vi "Get VISA_Class.vi"(8 "error in":errorcluster, 9 "Sequence Context In":refnum<k7>, 10 "Config path":path=path "C:/GitHub/OOP_Submodule EOL/Config/INI Config.ini", 11 "Instrument":string="DMM") -> (0 "error out":errorcluster, 2 "Class":string, 3 "VISA Resource":string)   [LabVIEW 2021]
uses:
  Controls/Instrument.ctl
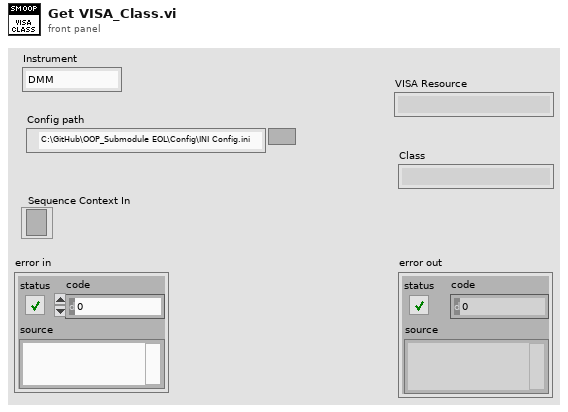
[diagram p1: front panel]
types:
  T1 = typedef "Instrument.ctl" = cluster{"Alias":string, "VISA Resource":string, "Class":string}
  T2 = typedef "MsgData.ctl" = cluster{"Message":string, "Data":variant}
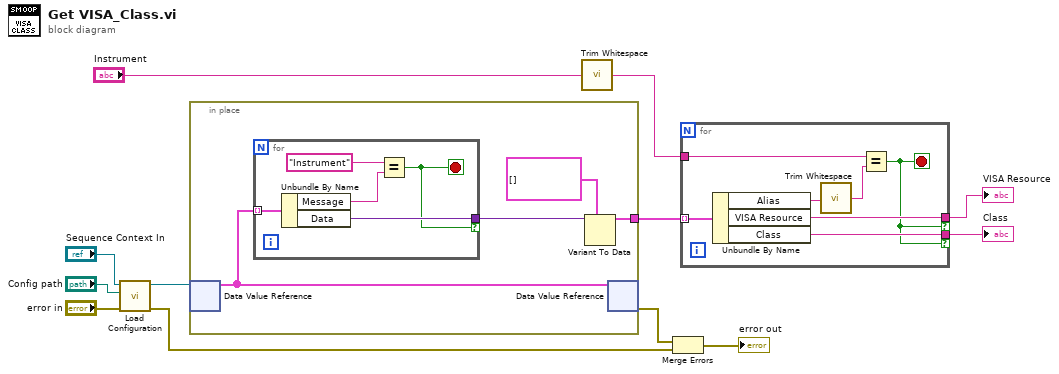
[diagram p0: block diagram]
diagram:
  n1 = call "Load Configuration.vi"("error in"="error in", "Config path"="Config path", "Sequence Context In"="Sequence Context In") -> ("error out"=w3:errorcluster, "Config DVR"=w8:refnum<data-value>)  [unwired: 7 in]
  n2 = in-place {
    in-place-border: [w13] -> w7
    n3 = in-place-dvr #1(w8) -> (w14:T2[])  [unwired: 1 out]
    n4 = for {
      tunnel: w14 -> [w21] mode=indexing
      tunnel: [w18] -> w16 if=w17
      stop <- w17 stop-if-true
      n5 = Unbundle By Name(w21) -> ("Message"=w20:string, "Data"=w18:variant)
      n6 = Equal?(x="Instrument" ("Name"), y=w20) -> (x = y?=w17:bool)
    }
    n7 = Variant To Data(type=T1[] [], Variant=w16) -> (data=w13:T1[])  [unwired: 1 in, 1 out]
    n8 = in-place-dvr #1(w14) -> (w6:errorcluster)  [unwired: 1 out]
  }
  n9 = call <vilib>:"Trim Whitespace.vi"("string"="Instrument") -> ("trimmed string"=w9:string)  [unwired: 1 in]
  n10 = Merge Errors(w6, w3) -> (→"error out":errorcluster)
  n11 = for {
    tunnel: w7 -> [w28] mode=indexing
    tunnel: w9 -> [w27]
    tunnel: [w26] -> w12 if=w24
    tunnel: [w25] -> w11 if=w24
    stop <- w24 stop-if-true
    n12 = Unbundle By Name(w28) -> ("Alias"=w23:string, "VISA Resource"=w26:string, "Class"=w25:string)
    n13 = call <vilib>:"Trim Whitespace.vi"("string"=w23) -> ("trimmed string"=w22:string)  [unwired: 1 in]
    n14 = Equal?(x=w27, y=w22) -> (x = y?=w24:bool)
  }
  "VISA Resource" <- w12
  "Class" <- w11
